vi "FTW-Benchmark-JSON.vi"() -> ()   [LabVIEW 2012]
uses:
  Core/src/JSON/FTW-JSON.lvclass
panel:
  out "Results":T1(array[cluster]) {"Elapsed Time" format="%.6fsec"}
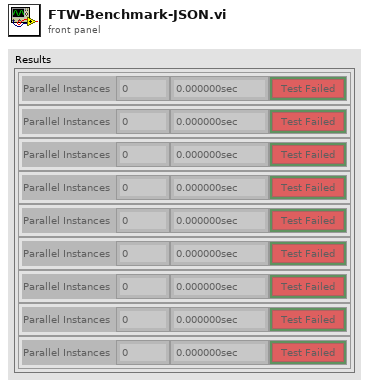
[diagram p1: front panel]
types:
  T1 = cluster{"Parallel Instances":i32, "Elapsed Time":dbl, bool}[]
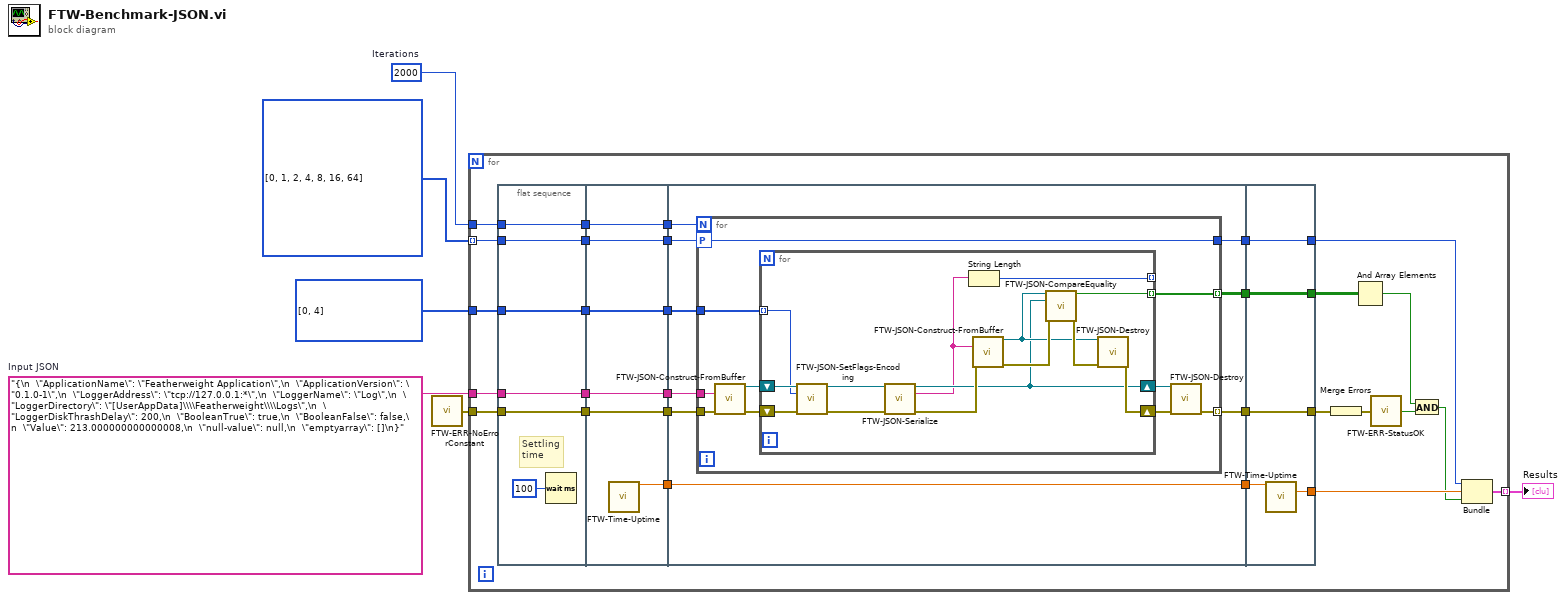
[diagram p0: block diagram]
diagram:
  w5 = "{\n  \"ApplicationName\": \"Featherweight Application\",\n  \"ApplicationVersion\": \"0.1.0-1\",\n  \"LoggerAddress\": \"tcp://127.0.0.1:*\",\n  \"LoggerName\": \"Log\",\n  \"LoggerDirectory\": \"[UserAppData]\\\\Featherweight\\\\Logs\",\n  \"LoggerDiskThrashDelay\": 200,\n  \"BooleanTrue\": true,\n  \"BooleanFalse\": false,\n  \"Value\": 213.000000000000008,\n  \"null-value\": null,\n  \"emptyarray\": []\n}"  # Input JSON
  w6 = 2000  # Iterations
  n1 = call "FTW-ERR-NoErrorConstant.vi"() -> ("no error"=w4:errorcluster)
  n2 = for {
    tunnel: w6 -> [w27]
    tunnel: w5 -> [w26]
    tunnel: w4 -> [w25]
    tunnel: i32[] [0, 4] -> [w24]
    tunnel: i32[] [0, 1, 2, 4, 8, 16, 64] -> [w20] mode=indexing
    tunnel: [w14] -> w1 mode=indexing
    n3 = flat-sequence {
      tunnel: w20 -> [w37]
      tunnel: w24 -> [w38]
      tunnel: w25 -> [w39]
      tunnel: w26 -> [w40]
      tunnel: w27 -> [w41]
      tunnel: [w41] -> w13
      tunnel: [w40] -> w12
      tunnel: [w39] -> w11
      tunnel: [w38] -> w10
      tunnel: [w37] -> w9
      tunnel: [w47] -> w35
      tunnel: [w46] -> w34
      tunnel: [w45] -> w33
      tunnel: [w44] -> w32
      tunnel: [w43] -> w31
      tunnel: [w42] -> w23
      tunnel: w13 -> [w47]
      tunnel: w12 -> [w46]
      tunnel: w11 -> [w45]
      tunnel: w10 -> [w44]
      tunnel: w9 -> [w42]
      tunnel: w35 -> [w56]
      tunnel: w34 -> [w48]
      tunnel: w33 -> [w54]
      tunnel: w32 -> [w52]
      tunnel: [w55] -> w30
      tunnel: [w53] -> w29
      tunnel: [w51] -> w28
      tunnel: w31 -> [w51]
      tunnel: w23 -> [w50]
      tunnel: [w49] -> w7
      tunnel: [w84] -> w19
      tunnel: [w85] -> w21
      tunnel: w30 -> [w85]
      tunnel: w29 -> [w84]
      tunnel: w28 -> [w83]
      tunnel: [w82] -> w22
      tunnel: [w81] -> w8
      tunnel: w7 -> [w81]
      frame #0 {
        # "Settling\ntime"
        n4 = Wait (ms)(milliseconds to wait=u32 100) -> ()  [unwired: 1 out]
      }
      frame #1 {
        n5 = call "FTW-Time-Uptime.vi"() -> ("Current Uptime"=w43:dbl)  [unwired: 13 in, 2 out]
      }
      frame #2 {
        n6 = for {
          N: w56 -> [_]
          tunnel: w48 -> [w64]
          tunnel: [w58] -> w53 mode=indexing
          tunnel: w52 -> [w59]
          workers-P: w50 -> [w57]
          tunnel: w54 -> [w66]
          tunnel: [w65] -> w55 mode=indexing
          tunnel: [w57] -> w49
          n7 = call "FTW-JSON-Construct-FromBuffer.vi"("JSON String (UTF-8)"=w64, "error in"=w66) -> ("JSON Object"=w60:refnum<class "FTW-JSON.lvclass">, "error out"=w61:errorcluster)  [unwired: 12 in]
          n8 = for {
            tunnel: w59 -> [w75] mode=indexing
            shift-right: [w72] -> w62
            shift-left: w60 -> [w76]
            shift-right: [w80] -> w63
            shift-left: w61 -> [w77]
            tunnel: [w71] -> w58 mode=indexing
            tunnel: [w69] -> _ mode=indexing
            n9 = call "FTW-JSON-SetFlags-Encoding.vi"("JSON Object"=w76, "Indent Spaces"=w75, "error in"=w77) -> ("JSON Object out"=w68:refnum<class "FTW-JSON.lvclass">, "error out"=w67:errorcluster)  [unwired: 11 in]
            n10 = call "FTW-JSON-Serialize.vi"("JSON Object"=w68, "error in"=w67) -> ("JSON Object out"=w72:refnum<class "FTW-JSON.lvclass">, "JSON String (UTF-8)"=w70:string, "error out"=w74:errorcluster)  [unwired: 11 in]
            n11 = String Length(string=w70) -> (length=w69:i32)
            n12 = call "FTW-JSON-Construct-FromBuffer.vi"("JSON String (UTF-8)"=w70, "error in"=w74) -> ("JSON Object"=w73:refnum<class "FTW-JSON.lvclass">, "error out"=w78:errorcluster)  [unwired: 12 in]
            n13 = call "FTW-JSON-CompareEquality.vi"("JSON Object"=w73, "JSON Object to Compare"=w72, "error in"=w78) -> ("Equal?"=w71:bool, "error out"=w79:errorcluster)  [unwired: 11 in]
            n14 = call "FTW-JSON-Destroy.vi"("JSON Object"=w73, "error in"=w79) -> ("error out"=w80:errorcluster)  [unwired: 13 in]
          }
          n15 = call "FTW-JSON-Destroy.vi"("JSON Object"=w62, "error in"=w63) -> ("error out"=w65:errorcluster)  [unwired: 13 in]
        }
      }
      frame #3 {
        n16 = call "FTW-Time-Uptime.vi"("Previous Uptime"=w83) -> ("Elapsed Time"=w82:dbl)  [unwired: 12 in, 2 out]
      }
    }
    n17 = Merge Errors(w21) -> (w18:errorcluster)
    n18 = And Array Elements(Boolean array=w19) -> (logical AND=w16:bool)
    n19 = call "FTW-ERR-StatusOK.vi"("error to check"=w18) -> ("Status OK?"=w17:bool)
    n20 = And(x=w16, y=w17) -> (x .and. y?=w15:bool)
    n21 = Bundle(w8, "Elapsed Time"=w22, w15) -> (w14:cluster{i32, "Elapsed Time":dbl, bool})  [unwired: 1 in]
  }
  "Results" <- w1
